vi "Arm Controller.vi"(1 "error in":errorcluster, 2 "Button7OnBothJostick1and2":bool, 3 "Input":dbl) -> (0 "error out":errorcluster)   [LabVIEW 2017]
uses:
  <vilib>/Rock Robotics/Network Tables/NT Write Number.vi
  Global Simulated Arm Pot.vi
  <vilib>/Rock Robotics/WPI/ThirdParty/Phoenix-LabVIEW/Motor Controller/Controls/CTRE_Phoenix_MotorControl_ControlMode.ctl
panel:
  out "Pot Value":dbl
  out "teleopMotorInput":dbl
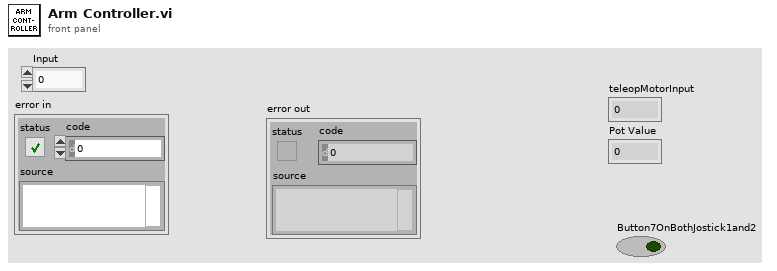
[diagram p1: front panel]
types:
  T1 = typedef "CTRE_Phoenix_MotorControl_ControlMode.ctl" = u16
  T2 = typedef "WPI_PotentiometerDevRef.ctl" = cluster{"DevStatus":errorcluster, "Analog Channel":T3, "Invert Output":bool}
  T3 = typedef "FPGA_AIChannel.ctl" = enum8{"AI 0", "AI 1", "AI 2", "AI 3", "AI MXP 0", "AI MXP 1", "AI MXP 2", "AI MXP 3", "Invalid"}
  T4 = typedef "WPI_MotorControlDeviceRef.ctl" = cluster{"DeviceStatus":errorcluster, "Type":T5, "PWM":cluster{"PWM Channel":T6, "DeadBand":T7}, "CAN":cluster{"Device Number":u8, "SetOutput VI Ref":variant, "GetOutput VI Ref":variant, "Enable VI Ref":variant, "Disable VI Ref":variant, "Data":variant}, "Invert":bool, "DIO PWM":cluster{"PWM \"Enable\" Channel":T6, "DIOChannel":T8, "PWM Rate":dbl}}
  T5 = typedef "WPI_MotorControlType.ctl" = enum16{"PWM", "CAN", "DIO PWM"}
  T6 = typedef "FPGA_DIOPWMChannel.ctl" = enum8{"PWM 0", "PWM 1", "PWM 2", "PWM 3", "PWM 4", "PWM 5", "PWM 6", "PWM 7", "PWM 8", "PWM 9", "PWM MXP 0", "PWM MXP 1", "PWM MXP 2", "PWM MXP 3", "PWM MXP 4", "PWM MXP 5", "PWM MXP 6", "PWM MXP 7", "PWM MXP 8", "PWM MXP 9", "Invalid"}
  T7 = typedef "WPI_PWMDeadband.ctl" = cluster{"Name":string, "maxPositivePwm":i32, "minPositivePwm":i32, "centerPwm":i32, "maxNegativePwm":i32, "minNegativePwm":i32, "angularRange":u16}
  T8 = typedef "FPGA_DIOChannel.ctl" = enum8{"DIO 0", "DIO 1", "DIO 2", "DIO 3", "DIO 4", "DIO 5", "DIO 6", "DIO 7", "DIO 8", "DIO 9", "DIO MXP 0", "DIO MXP 1", "DIO MXP 2", "DIO MXP 3", "DIO MXP 4", "DIO MXP 5", "DIO MXP 6", "DIO MXP 7", "DIO MXP 8", "DIO MXP 9", "DIO MXP 10", "DIO MXP 11", "DIO MXP 12", "DIO MXP 13", "DIO MXP 14", "DIO MXP 15", "SPI Port CS1", "SPI Port CS2", "SPI Port CS3", "SPI Port MISO", "SPI Port MOSI", "Invalid"}
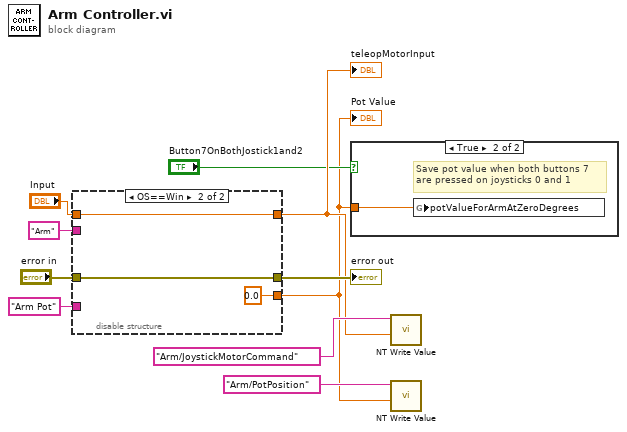
[diagram p0: block diagram]
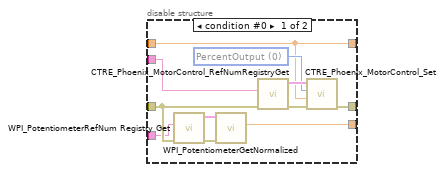
[diagram p3: hidden frame]
diagram:
  n1 = disable-structure shown="OS==Win" {
    disable-tunnel: "Arm" ("Motor ID") -> [w21 _]
    disable-tunnel: "Input" -> [w16 w23]
    disable-tunnel: [w17 w24] -> w7
    disable-tunnel: "error in" -> [w13 w24]
    disable-tunnel: [w16 w23] -> w5
    disable-tunnel: [w12 0.0 ("Normalized Value")] -> w1
    disable-tunnel: "Arm Pot" ("refnum name") -> [w11 _]
    frame condition #0 {
      w19 = T1 0 items=["PercentOutput"=0, "Position"=1, "Velocity"=2, "Current"=3, "Follower"=5, "MotionProfile"=6, "MotionMagic"=7, "MotionMagicArc"=8, "MotionProfileArc"=10, "Disabled"=15] ("Control Mode")
      n2 = call <vilib>:"WPI_PotentiometerRefNum Registry Get.vi"("error in (no error)"=w13, "refnum name"=w11) -> ("error out"=w14:errorcluster, "PotDevRef"=w15:T2)  [unwired: 8 in]
      n3 = call <vilib>:"WPI_PotentiometerGetNormalized.vi"("error in"=w14, "PotDevRef"=w15) -> ("Normalized Value"=w12:dbl)  [unwired: 7 in, 2 out]
      n4 = call <vilib>:"CTRE_Phoenix_MotorControl_RefNumRegistryGet.vi"("error in (no error)"=w13, "refnum name"=w21) -> ("error out"=w18:errorcluster, "PhoenixMotorControlDevRef"=w20:T4)  [unwired: 8 in]
      n5 = call <vilib>:"CTRE_Phoenix_MotorControl_Set.vi"("error in (no error)"=w18, "Output"=w16, "Control Mode"=w19, "PhoenixMotorControlDevRef"=w20) -> ("error out"=w17:errorcluster)  [unwired: 6 in, 1 out]
    }
    frame condition #1 (active) {
    }
  }
  "error out" <- w7
  "teleopMotorInput" <- w5
  "Pot Value" <- w1
  n6 = case shown="True" "Button7OnBothJostick1and2" {
    tunnel: w1 -> [_ w25]
    frame False {
    }
    frame True {
      # "Save pot value when both buttons 7\nare pressed on joysticks 0 and 1"
      n7 = global write "Global Simulated Arm Pot.vi" "potValueForArmAtZeroDegrees"(w25) -> ()
    }
  }
  n8 = call-poly <vilib>:"NT Write Value.vi"("Numeric"=w5, "Name"="Arm/JoystickMotorCommand") -> ()  [unwired: 9 in, 1 out]
  n9 = call-poly <vilib>:"NT Write Value.vi"("Numeric"=w1, "Name"="Arm/PotPosition") -> ()  [unwired: 9 in, 1 out]
